vi "ArchivosProfesor.vi"() -> ()   [LabVIEW 2023]
panel:
  out "text":string
  out "error out":errorcluster
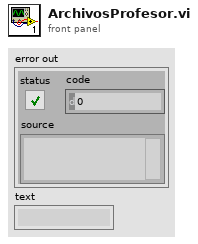
[diagram p1: front panel]
types:
  T1 = enum16{"open", "replace", "create", "open or create", "replace or create", "replace or create with confirmation"}
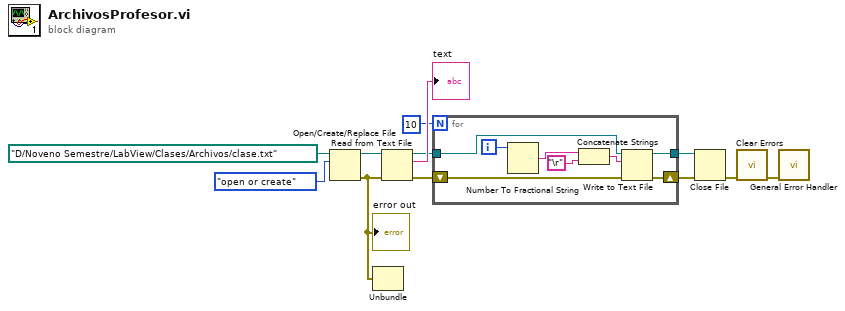
[diagram p0: block diagram]
diagram:
  n1 = Open/Create/Replace File(file path (use dialog)=path "D:/Noveno Semestre/LabView/Clases/Archivos/clase.txt", operation (0:open)=T1."open or create") -> (refnum out=w11:refnum<file>, error out=w8:errorcluster)  [unwired: 4 in, 1 out]
  "error out" <- w8
  n2 = Unbundle(w8) -> ()  [unwired: 3 out]
  n3 = Read from Text File(file (use dialog)=w11, error in=w8) -> (refnum out=w5:refnum<file>, text=→"text":string, error out=w3:errorcluster)  [unwired: 2 in, 1 out]
  n4 = for {
    N: 10 -> [_]
    tunnel: w5 -> [w20]
    tunnel: [w19] -> w4
    shift-right: [w17] -> w2
    shift-left: w3 -> [w18]
    i -> [w16]
    n5 = Number To Fractional String(number=w16) -> (F-format string=w15:string)  [unwired: 3 in]
    n6 = Concatenate Strings(w15, "\r") -> (w13:string)
    n7 = Write to Text File(file (use dialog)=w20, text=w13, error in=w18) -> (refnum out=w19:refnum<file>, error out=w17:errorcluster)  [unwired: 1 in, 1 out]
  }
  n8 = Close File(refnum=w4, error in=w2) -> (error out=w6:errorcluster)  [unwired: 1 out]
  n9 = call <vilib>:"Clear Errors.vi"("error in (no error)"=w6) -> ("error out"=w9:errorcluster)  [unwired: 5 in, 1 out]
  n10 = call <vilib>:"General Error Handler.vi"("error in (no error)"=w9) -> ()  [unwired: 10 in, 5 out]
